vi "Pololu.Dual Servo Controller.vi"() -> ()   [LabVIEW 2018]
uses:
  <vilib>/KATE/Queues/Q.Element.ctl
  Dual Servo Manager Class/PololuCtrl.lvclass
  Pololu.Commands.ctl
  <vilib>/KATE/Queues/Queue Utils.lvlib
panel:
  in  "Tab Control":enum32{"Operate", "Maint"}(tab)
  out "Connected":bool
  out "error":errorcluster
  in  "Connect":bool
  in  "Disconnect":bool
  out "COM Port":string
  in  "Set Speed":bool
  in  "Set Accel":bool
  in  "Deg/Sec":dbl
  in  "Deg/Sec/Sec":dbl
  in  "Chan":u8
  in  "Set Pos":bool
  in  "Track Ctrl":bool
  in  "Set Pos (Deg)":dbl(slide) max=270.0 scale=0.0..270.0
  out "Cmd us":dbl
  out "Cmd units":u16
  out "Stored Pos":dbl[](array[numeric])
  in  "Store Pos":bool
  in  "Pos ID":i32
  in  "Go To Pos":bool
  in  "Get Pos":bool
  out "Read Pos (Units)":u16 max=270
  in  "Get Errors":bool
  out "Read Errors":u16 max=270 format="%016b"
  in  "Get Moving":bool
  out "Moving":bool
  in  "Master Q":refnum<queue>
  in  "Min us":dbl
  in  "Min deg":dbl
  in  "Max deg":dbl=270.0
  in  "Max us":dbl=2500.0
  in  "VID":string="1FFB"
  in  "PID":string="0089"
  in  "Q Name":string
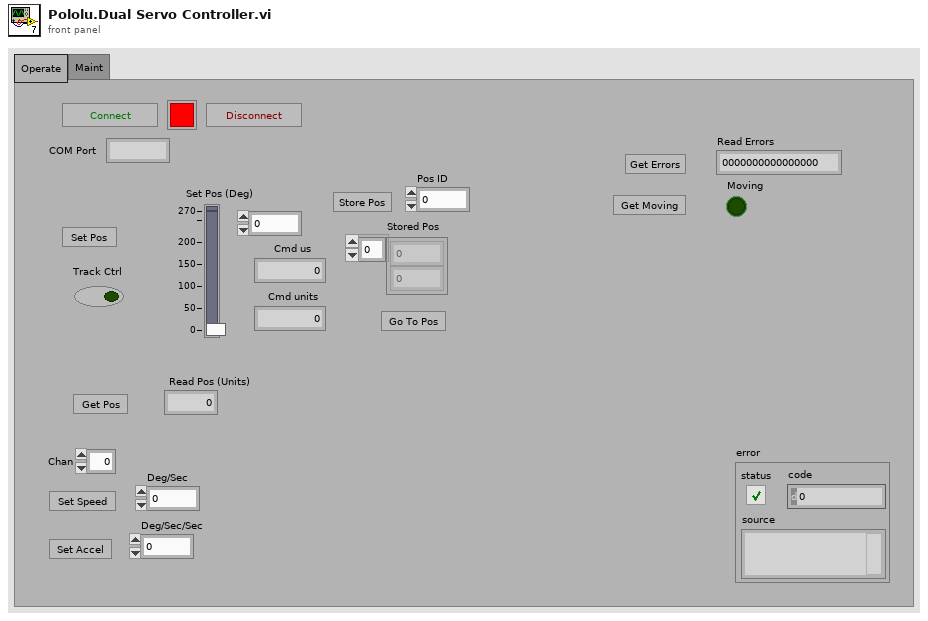
[diagram p1: front panel]
types:
  T1 = typedef "Pololu.Commands.ctl" = enum16{"Set Pos", "Set Speed", "Set Accel", "Get Pos", "Get Mov Status", "Get Errors"}
  T2 = cluster{"Pololu":refnum<class "PololuCtrl.lvclass">}
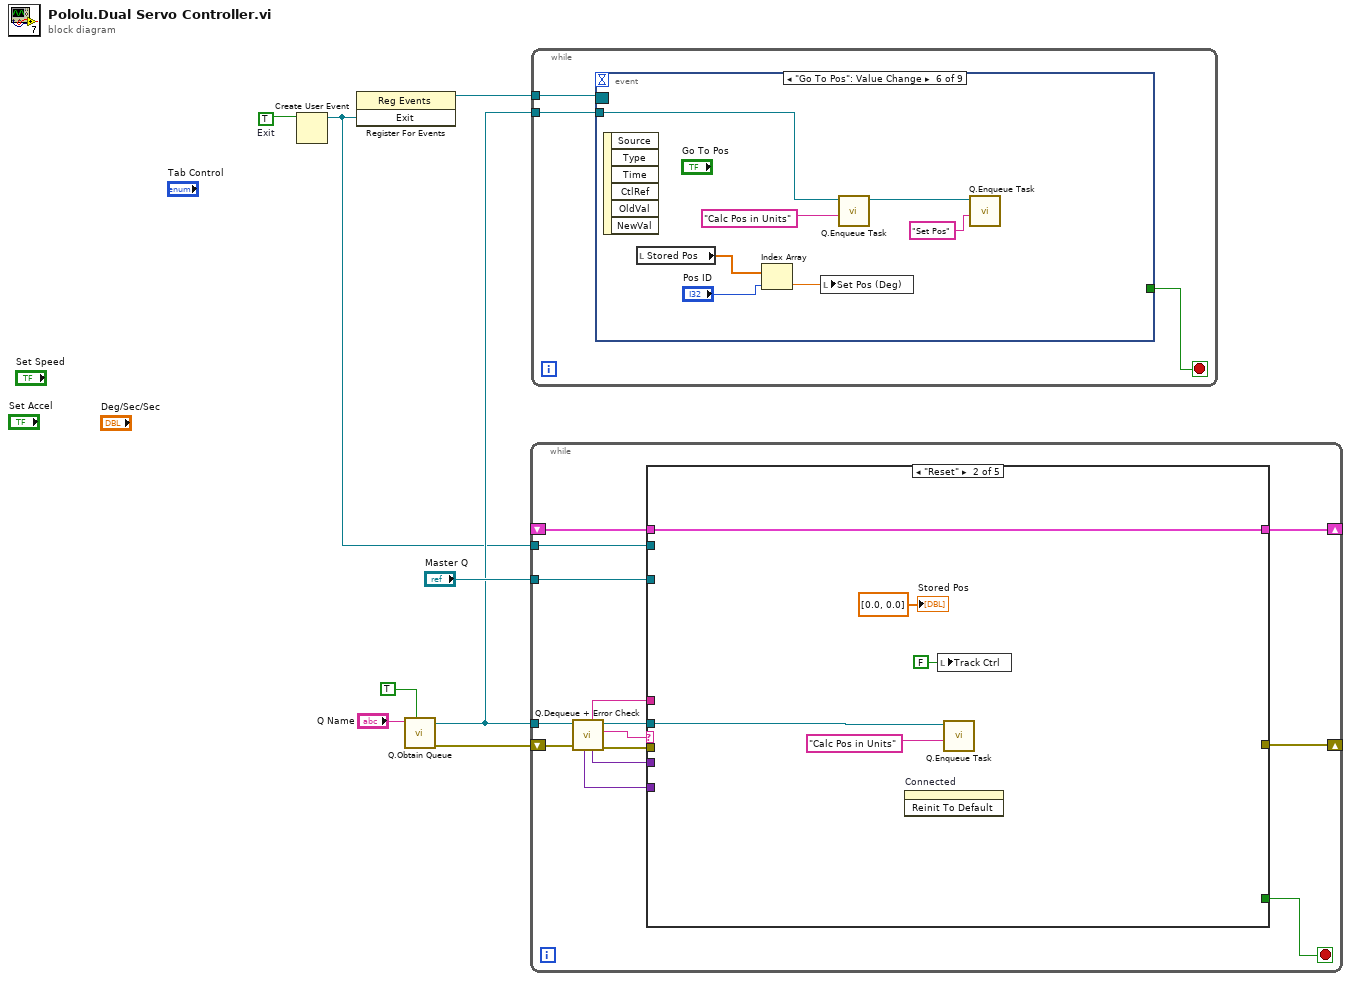
[diagram p0: block diagram]
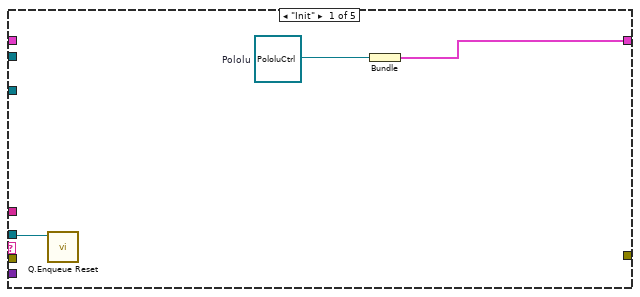
[diagram p2: hidden frame]
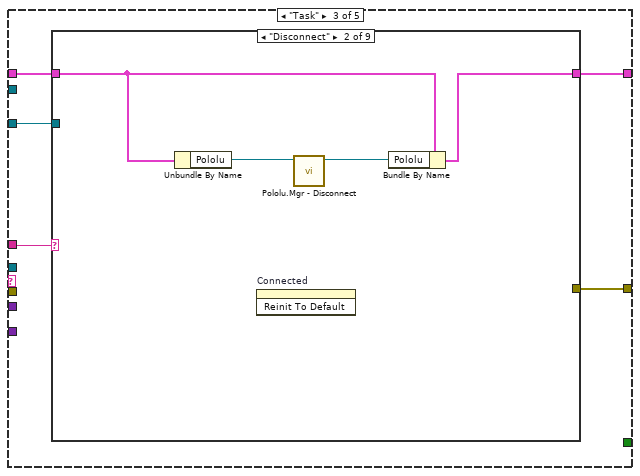
[diagram p3: hidden frame]
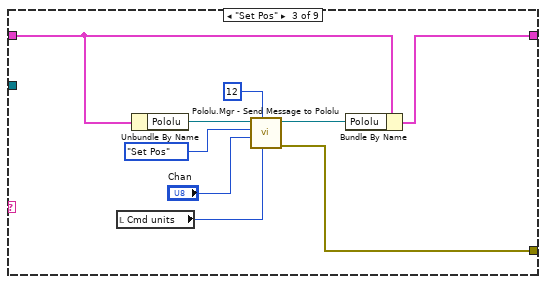
[diagram p5: hidden frame]
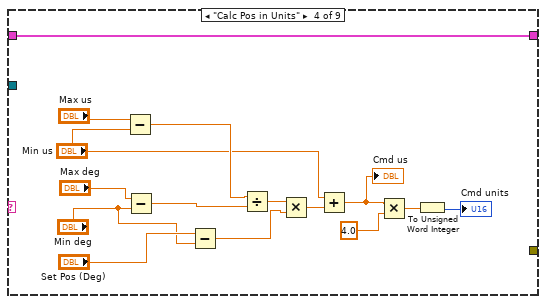
[diagram p6: hidden frame]
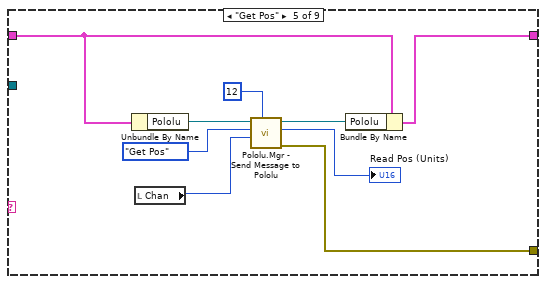
[diagram p7: hidden frame]
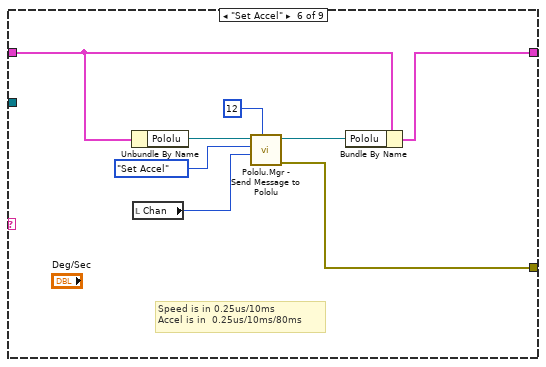
[diagram p8: hidden frame]
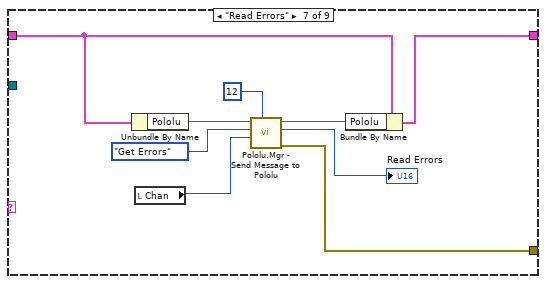
[diagram p9: hidden frame]
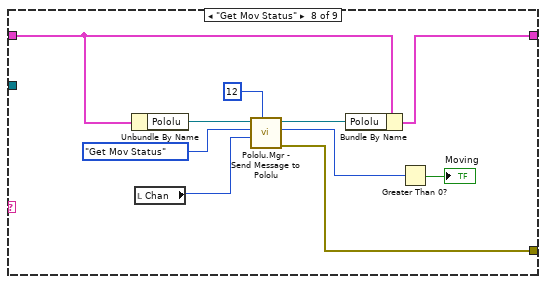
[diagram p10: hidden frame]
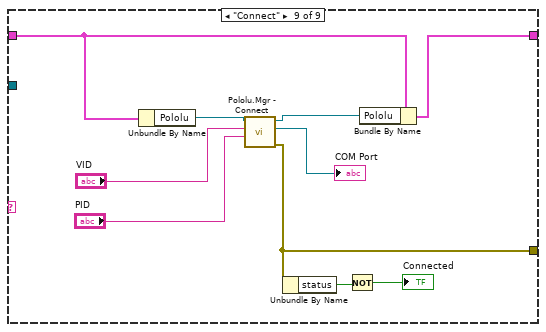
[diagram p11: hidden frame]
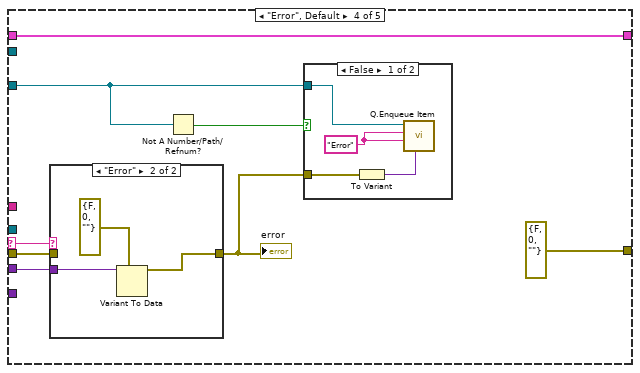
[diagram p12: hidden frame]
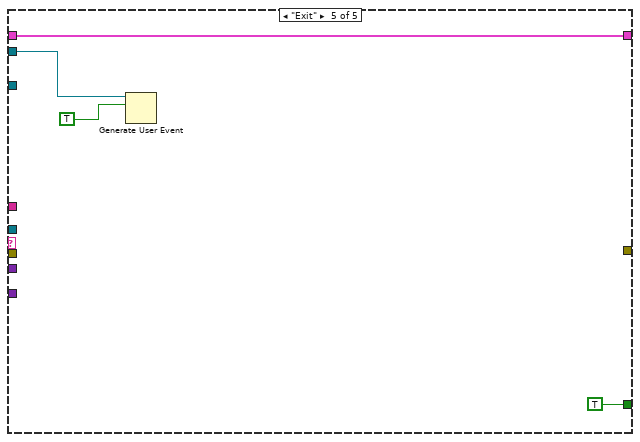
[diagram p15: hidden frame]
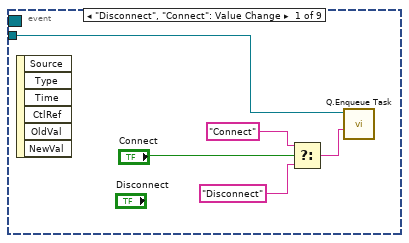
[diagram p16: hidden frame]
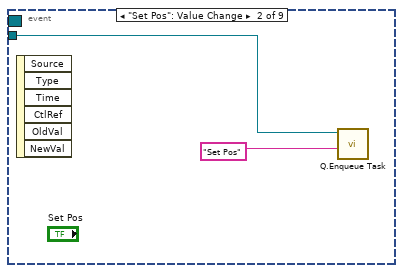
[diagram p17: hidden frame]
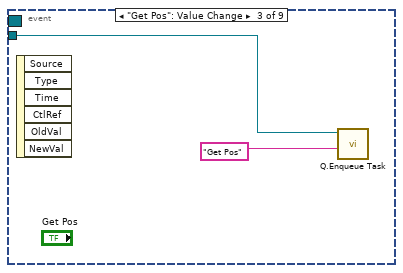
[diagram p18: hidden frame]
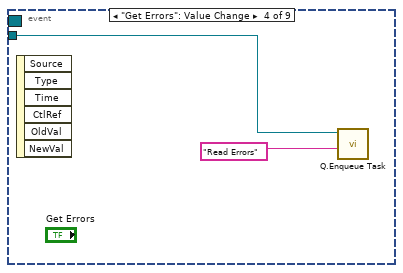
[diagram p19: hidden frame]
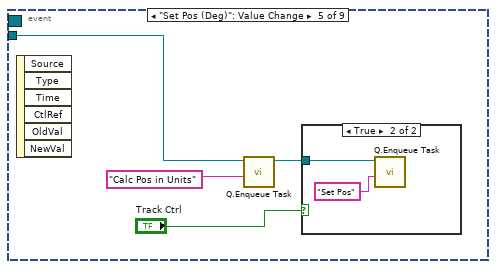
[diagram p20: hidden frame]
diagram:
  w3 = TRUE  # Exit
  n1 = Create User Event(user event datatype=w3) -> (user event=w2:refnum<user-event>)  [unwired: 1 in, 1 out]
  n2 = register-events(w2) -> (reference out=w1:refnum<event-registration>)  [unwired: 2 in, 1 out]
  n3 = call <vilib>:"Q.Obtain Queue.vi"("Enqueue Init"=TRUE, "Q Name"="Q Name") -> ("error out"=w8:errorcluster, "Q Out"=w4:refnum<queue>)  [unwired: 7 in, 1 out]
  n4 = while {
    tunnel: w4 -> [w22]
    shift-right: [w12] -> _
    shift-left: w8 -> [w21]
    shift-right: [w10] -> _
    shift-left: _ -> [w15]
    tunnel: "Master Q" -> [w14]
    tunnel: w2 -> [w9]
    stop <- w11 stop-if-true
    n5 = call <vilib>:"Q.Dequeue + Error Check.vi"("Error In"=w21, "Q In"=w22) -> ("error out"=w13:errorcluster, "Cmd"=w20:string, "Q Out"=w19:refnum<queue>, "Data1"=w17:variant, "Sub"=w18:string, "Data2"=w16:variant)  [unwired: 4 in]
    n6 = case shown="\"Reset\"" w20 {
      selector: w20 -> [_ _ _ w118 _]
      tunnel: w19 -> [w23 w28 _ _ _]
      tunnel: w18 -> [_ _ w35 _ _]
      tunnel: w17 -> [_ _ _ w116 _]
      tunnel: w16 -> [_ _ _ _ _]
      tunnel: w15 -> [_ w30 w33 w114 w129]
      tunnel: w14 -> [_ _ w34 w112 _]
      tunnel: w13 -> [_ _ _ w117 _]
      tunnel: [_ _ w31 errorcluster {"status"=FALSE, "code"=0, "source"=""} ("error") _] -> w12
      tunnel: [_ _ _ _ TRUE] -> w11
      tunnel: [w24 w30 w32 w114 w129] -> w10
      tunnel: w9 -> [_ _ _ _ w127]
      frame "Init" {
        w25 = refnum<class "PololuCtrl.lvclass"> refnum  # Pololu
        n7 = call <vilib>:"Q.Enqueue Reset.vi"("Q In"=w23) -> ()  [unwired: 9 in, 2 out]
        n8 = Bundle("Pololu"=w25) -> (w24:T2)  [unwired: 1 in]
      }
      frame "Reset" {
        n9 = invoke on="Connected" class="Bool (strict)" method="Reinit To Default"() -> ()  [unwired: 3 in, 3 out]
        n10 = local write "Track Ctrl"(FALSE ("Track Ctrl")) -> ()
        n11 = call <vilib>:"Q.Enqueue Task.vi"("Task Name"="Calc Pos in Units", "Q In"=w28) -> ()  [unwired: 8 in, 2 out]
        "Stored Pos" <- dbl[] [0.0, 0.0] ("Stored Pos")
      }
      frame "Task" {
        n12 = case shown="\"Disconnect\"" w35 {
          tunnel: w34 -> [_ _ _ _ _ _ _ _ _]
          tunnel: w33 -> [w36 w40 w49 w64 w73 w81 w90 w100 w110]
          tunnel: [w36 w39 w48 w64 w72 w80 w89 w99 w109] -> w32
          tunnel: [_ _ w42 _ w67 w75 w84 w94 w103] -> w31
          frame Default {
          }
          frame "Disconnect" {
            n13 = Unbundle By Name(w40) -> ("Pololu"=w38:refnum<class "PololuCtrl.lvclass">)
            n14 = invoke on="Connected" class="Bool (strict)" method="Reinit To Default"() -> ()  [unwired: 3 in, 3 out]
            n15 = call "Pololu.Mgr - Disconnect.vi"("PololuCtrl in"=w38) -> ("PololuCtrl out"=w37:refnum<class "PololuCtrl.lvclass">)  [unwired: 9 in, 1 out]
            n16 = Bundle By Name(cluster=w40, "Pololu"=w37) -> (w39:T2)
          }
          frame "Set Pos" {
            n17 = local read "Cmd units"() -> (w41:u16)
            n18 = Unbundle By Name(w49) -> ("Pololu"=w47:refnum<class "PololuCtrl.lvclass">)
            n19 = call "Pololu.Mgr - Send Message to Pololu.vi"("Value"=w41, "Device"=u8 12, "Channel"="Chan", "Command"=Pololu.Commands."Set Pos", "PololuCtrl in"=w47) -> ("error out"=w42:errorcluster, "PololuCtrl out"=w46:refnum<class "PololuCtrl.lvclass">)  [unwired: 4 in, 1 out]
            n20 = Bundle By Name(cluster=w49, "Pololu"=w46) -> (w48:T2)
          }
          frame "Calc Pos in Units" {
            n21 = Subtract(x="Max us", y="Min us") -> (x-y=w58:dbl)
            n22 = Subtract(x="Max deg", y="Min deg") -> (x-y=w57:dbl)
            n23 = Subtract(x="Set Pos (Deg)", y="Min deg") -> (x-y=w55:dbl)
            n24 = Divide(x=w58, y=w57) -> (x/y=w56:dbl)
            n25 = Multiply(x=w56, y=w55) -> (x*y=w54:dbl)
            n26 = Add(x="Min us", y=w54) -> (x+y=w52:dbl)
            "Cmd us" <- w52
            n27 = Multiply(x=w52, y=4.0) -> (x*y=w51:dbl)
            n28 = To Unsigned Word Integer(number=w51) -> (unsigned 16bit integer=→"Cmd units":u16)
          }
          frame "Get Pos" {
            n29 = Unbundle By Name(w73) -> ("Pololu"=w71:refnum<class "PololuCtrl.lvclass">)
            n30 = local read "Chan"() -> (w66:u8)
            n31 = call "Pololu.Mgr - Send Message to Pololu.vi"("Device"=u8 12, "Channel"=w66, "Command"=Pololu.Commands."Get Pos", "PololuCtrl in"=w71) -> ("error out"=w67:errorcluster, "Response"=→"Read Pos (Units)":u16, "PololuCtrl out"=w70:refnum<class "PololuCtrl.lvclass">)  [unwired: 5 in]
            n32 = Bundle By Name(cluster=w73, "Pololu"=w70) -> (w72:T2)
          }
          frame "Set Accel" {
            # "Speed is in 0.25us/10ms\nAccel is in  0.25us/10ms/80ms"
            n33 = Unbundle By Name(w81) -> ("Pololu"=w79:refnum<class "PololuCtrl.lvclass">)
            n34 = local read "Chan"() -> (w74:u8)
            n35 = call "Pololu.Mgr - Send Message to Pololu.vi"("Device"=u8 12, "Channel"=w74, "Command"=Pololu.Commands."Set Accel", "PololuCtrl in"=w79) -> ("error out"=w75:errorcluster, "PololuCtrl out"=w78:refnum<class "PololuCtrl.lvclass">)  [unwired: 5 in, 1 out]
            n36 = Bundle By Name(cluster=w81, "Pololu"=w78) -> (w80:T2)
          }
          frame "Read Errors" {
            n37 = Unbundle By Name(w90) -> ("Pololu"=w88:refnum<class "PololuCtrl.lvclass">)
            n38 = local read "Chan"() -> (w83:u8)
            n39 = call "Pololu.Mgr - Send Message to Pololu.vi"("Device"=u8 12, "Channel"=w83, "Command"=Pololu.Commands."Get Errors", "PololuCtrl in"=w88) -> ("error out"=w84:errorcluster, "Response"=→"Read Errors":u16, "PololuCtrl out"=w87:refnum<class "PololuCtrl.lvclass">)  [unwired: 5 in]
            n40 = Bundle By Name(cluster=w90, "Pololu"=w87) -> (w89:T2)
          }
          frame "Get Mov Status" {
            n41 = Unbundle By Name(w100) -> ("Pololu"=w98:refnum<class "PololuCtrl.lvclass">)
            n42 = local read "Chan"() -> (w93:u8)
            n43 = call "Pololu.Mgr - Send Message to Pololu.vi"("Device"=u8 12, "Channel"=w93, "Command"=Pololu.Commands."Get Mov Status", "PololuCtrl in"=w98) -> ("error out"=w94:errorcluster, "Response"=w92:u16, "PololuCtrl out"=w97:refnum<class "PololuCtrl.lvclass">)  [unwired: 5 in]
            n44 = Bundle By Name(cluster=w100, "Pololu"=w97) -> (w99:T2)
            n45 = Greater Than 0?(x=w92) -> (x > 0?=→"Moving":bool)
          }
          frame "Connect" {
            n46 = Unbundle By Name(w110) -> ("Pololu"=w108:refnum<class "PololuCtrl.lvclass">)
            n47 = call "Pololu.Mgr - Connect.vi"("PID"="PID", "VID"="VID", "PololuCtrl in"=w108) -> ("error out"=w103:errorcluster, "Com Port"=→"COM Port":refnum<visa-resource-name>, "PololuCtrl out"=w107:refnum<class "PololuCtrl.lvclass">)  [unwired: 6 in]
            n48 = Unbundle By Name(w103) -> ("status"=w102:bool)
            n49 = Not(x=w102) -> (.not. x?=→"Connected":bool)
            n50 = Bundle By Name(cluster=w110, "Pololu"=w107) -> (w109:T2)
          }
        }
      }
      frame "Error", Default {
        n51 = case shown="\"Error\"" w118 {
          tunnel: w117 -> [w123 _]
          tunnel: [w123 w125] -> w111
          tunnel: w116 -> [_ w126]
          frame Default {
          }
          frame "Error" {
            n52 = Variant To Data(type=errorcluster {"status"=FALSE, "code"=0, "source"=""} ("error"), Variant=w126) -> (data=w125:errorcluster)  [unwired: 1 in, 1 out]
          }
        }
        "error" <- w111
        n53 = Not A Number/Path/Refnum?(number/path/refnum=w112) -> (NaN/Path/Refnum?=w113:bool)
        n54 = case shown="False" w113 {
          tunnel: w112 -> [w122 _]
          tunnel: w111 -> [w119 _]
          frame False {
            w121 = "Error" ("Cmd")
            n55 = To Variant(anything=w119) -> (Variant=w120:variant)
            n56 = call <vilib>:"Q.Enqueue Item.vi"("Data1"=w120, "Sub"=w121, "Cmd"=w121, "Q In"=w122) -> ()  [unwired: 6 in, 2 out]
          }
          frame True {
          }
        }
      }
      frame "Exit" {
        n57 = Generate User Event(user event=w127, event data cluster=TRUE) -> ()  [unwired: 2 in, 2 out]
      }
    }
  }
  n58 = while {
    tunnel: w4 -> [w133]
    tunnel: w1 -> [w132]
    stop <- w131 stop-if-true
    n59 = event shown="[5] \"Go To Pos\": Value Change" {
      selector: w132 -> [_ _ _ _ _ _ _ _ _]
      dyn-events: _ -> [_ _ _ _ _ _ _ _ _]
      timeout: _ -> [_ _ _ _ _ _ _ _ _]
      tunnel: w133 -> [w138 w140 w142 w144 w147 w153 _ w163 w166]
      tunnel: [_ _ _ _ _ _ _ _ TRUE] -> w131
      event "Disconnect", "Connect": Value Change {
        n60 = event-data() -> ()  [unwired: 1 in, 6 out]
        n61 = Select(t="Connect", s="Connect", f="Disconnect") -> (s? t:f=w135:string)
        n62 = call <vilib>:"Q.Enqueue Task.vi"("Task Name"=w135, "Q In"=w138) -> ()  [unwired: 8 in, 2 out]
      }
      event "Set Pos": Value Change {
        n63 = event-data() -> ()  [unwired: 1 in, 6 out]
        n64 = call <vilib>:"Q.Enqueue Task.vi"("Task Name"="Set Pos", "Q In"=w140) -> ()  [unwired: 8 in, 2 out]
      }
      event "Get Pos": Value Change {
        n65 = event-data() -> ()  [unwired: 1 in, 6 out]
        n66 = call <vilib>:"Q.Enqueue Task.vi"("Task Name"="Get Pos", "Q In"=w142) -> ()  [unwired: 8 in, 2 out]
      }
      event "Get Errors": Value Change {
        n67 = event-data() -> ()  [unwired: 1 in, 6 out]
        n68 = call <vilib>:"Q.Enqueue Task.vi"("Task Name"="Read Errors", "Q In"=w144) -> ()  [unwired: 8 in, 2 out]
      }
      event "Set Pos (Deg)": Value Change {
        n69 = event-data() -> ()  [unwired: 1 in, 6 out]
        n70 = call <vilib>:"Q.Enqueue Task.vi"("Task Name"="Calc Pos in Units", "Q In"=w147) -> ("Q Out"=w146:refnum<queue>)  [unwired: 8 in, 1 out]
        n71 = case shown="True" "Track Ctrl" {
          tunnel: w146 -> [_ w150]
          frame False {
          }
          frame True {
            n72 = call <vilib>:"Q.Enqueue Task.vi"("Task Name"="Set Pos", "Q In"=w150) -> ()  [unwired: 8 in, 2 out]
          }
        }
      }
      event "Go To Pos": Value Change {
        n73 = event-data() -> ()  [unwired: 1 in, 6 out]
        n74 = local read "Stored Pos"() -> (w156:dbl[])
        n75 = Index Array(array=w156, index="Pos ID") -> (element=w154:dbl)
        n76 = local write "Set Pos (Deg)"(w154) -> ()
        n77 = call <vilib>:"Q.Enqueue Task.vi"("Task Name"="Calc Pos in Units", "Q In"=w153) -> ("Q Out"=w152:refnum<queue>)  [unwired: 8 in, 1 out]
        n78 = call <vilib>:"Q.Enqueue Task.vi"("Task Name"="Set Pos", "Q In"=w152) -> ()  [unwired: 8 in, 2 out]
      }
      event "Store Pos": Value Change {
        n79 = event-data() -> ()  [unwired: 1 in, 6 out]
        n80 = local read "Set Pos (Deg)"() -> (w158:dbl)
        n81 = local read "Pos ID"() -> (w159:i32)
        n82 = local read "Stored Pos"() -> (w161:dbl[])
        n83 = Replace Array Subset(array=w161, new element=w158, index=w159) -> (w160:dbl[])
        n84 = local write "Stored Pos"(w160) -> ()
      }
      event "Get Moving": Value Change {
        n85 = event-data() -> ()  [unwired: 1 in, 6 out]
        n86 = call <vilib>:"Q.Enqueue Task.vi"("Task Name"="Get Mov Status", "Q In"=w163) -> ()  [unwired: 8 in, 2 out]
      }
      event Panel Close? {
        n87 = event-data() -> ()  [unwired: 1 in, 4 out]
        n88 = call <vilib>:"Q.Enqueue Exit.vi"("Q In"=w166) -> ()  [unwired: 9 in, 2 out]
        n89 = event-data("Discard?"=TRUE) -> ()  [unwired: 1 in, 1 out]
      }
    }
  }
